vi "Test Basic Function 1.vi"() -> ()   [LabVIEW 2014]
uses:
  <vilib>/Aledyne-TSXperts/Arduino Compatible Compiler for LabVIEW/addons/Arduino Math/Arduino Math.lvlib
panel:
  out "result":sgl
  out "Error Out":errorcluster
  in  "Error In":errorcluster
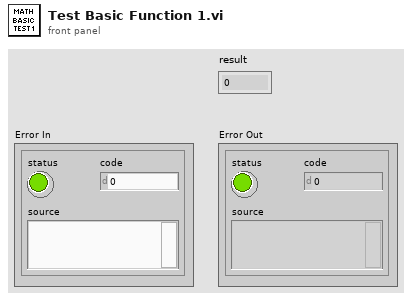
[diagram p1: front panel]
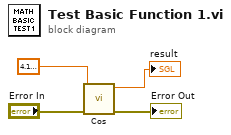
[diagram p0: block diagram]
diagram:
  n1 = call <vilib>:"Cos.vi"("Error In"="Error In", "x"=sgl 4.2) -> ("Error Out"=→"Error Out":errorcluster, "result"=→"result":sgl)  [unwired: 8 in]
